vi "GEA3 Decode Relay States.vi"(10 "ERD Relay Value":u32 format="%x", 11 "T1 Temp":dbl) -> (1 "Lower Element (0x4033)":bool, 2 "Upper Element (0x4033)":bool, 3 "Compressor (0x4033)":bool, 4 "Fan (0x4033)":bool)   [LabVIEW 2019]
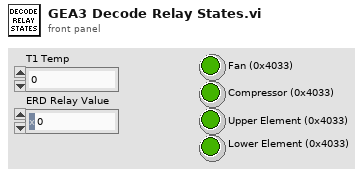
[diagram p1: front panel]
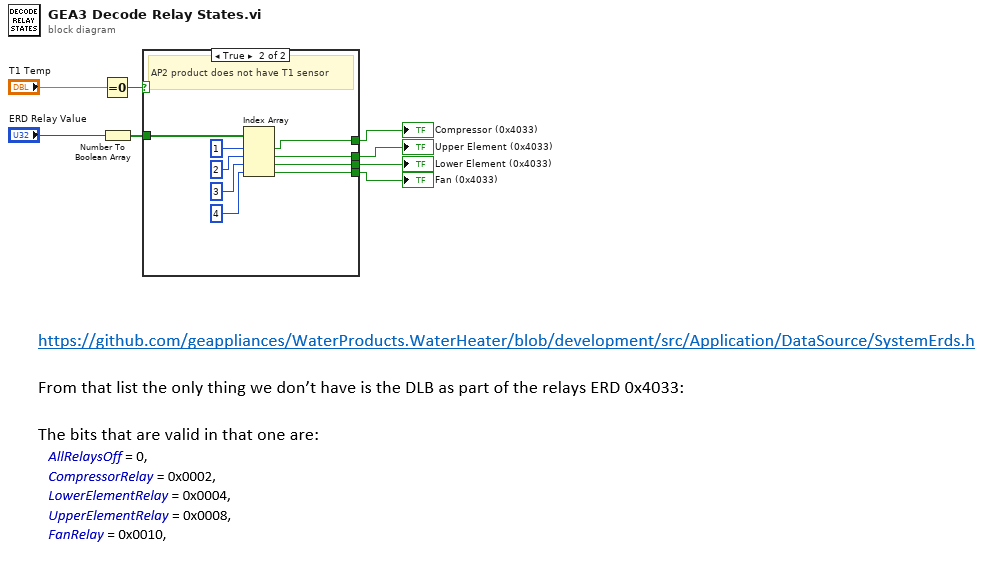
[diagram p0: block diagram]
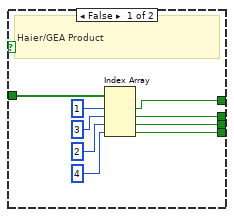
[diagram p2: hidden frame]
diagram:
  n1 = Equal To 0?(x="T1 Temp") -> (x = 0?=w8:bool)
  n2 = Number To Boolean Array(number="ERD Relay Value") -> (Boolean array=w5:bool[])
  n3 = case shown="True" w8 {
    tunnel: [w9 w22] -> w1
    tunnel: [w10 w23] -> w2
    tunnel: [w11 w24] -> w3
    tunnel: [w12 w25] -> w4
    tunnel: w5 -> [w17 w26]
    frame False {
      # "Haier/GEA Product"
      n4 = Index Array(array=w17, index #1=1 ("index"), index #2=3 ("index"), index #3=2 ("index"), index #4=4 ("index")) -> (element #1=w12:bool, element #2=w11:bool, element #3=w10:bool, element #4=w9:bool)
    }
    frame True {
      # "AP2 product does not have T1 sensor"
      n5 = Index Array(array=w26, index #1=1 ("index"), index #2=2 ("index"), index #3=3 ("index"), index #4=4 ("index")) -> (element #1=w25:bool, element #2=w24:bool, element #3=w23:bool, element #4=w22:bool)
    }
  }
  "Compressor (0x4033)" <- w4
  "Upper Element (0x4033)" <- w3
  "Lower Element (0x4033)" <- w2
  "Fan (0x4033)" <- w1
